vi "_Attenuator Tree.vi"   [LabVIEW 2011]
uses:
  LIB/Attenuator Version.vi
panel:
  # "See Diagram"
types:
  T1 = typedef "OGAB Version.ctl" = cluster{"Version":string, "Build Number":u32, "Build Date/Time":dbl}
  T2 = typedef "Field Record.ctl" = cluster{"ixField":i32, "iSequenceOrder":i32, "sxFieldId":string, "sxSequenceId":string, "sDisplayName":string, "sValue":string, "sUnits":string, "nDataType":T3, "nNextItem":T4, "fSystem":bool, "fSystemValue":bool, "fRequired":bool, "fSetAtTest":bool, "fTestField":bool, "fDeleted":bool, "fIndexed":bool, "fFreeList":bool}
  T3 = typedef "Field DataTypes.ctl" = enum32{"text", "numeric", "list", "timestamp", "boolean"}
  T4 = typedef "Field NextItem.ctl" = enum32{"Reset", "Retain", "Auto-Increment"}
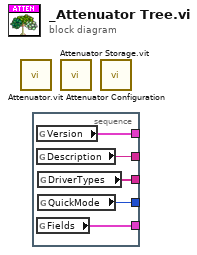
[diagram p0: block diagram]
diagram:
  n1 = call "Attenuator.vit"() -> ()  [unwired: 4 in, 8 out]
  n2 = stacked-sequence {
    tunnel: [w5] -> _
    tunnel: [w4] -> _
    tunnel: [w3] -> _
    tunnel: [w2] -> _
    tunnel: [w1] -> _
    frame #0 {
      n3 = global read "Attenuator Version.vi" "Version"() -> (w5:T1)
      n4 = global read "Attenuator Version.vi" "Description"() -> (w4:string)
      n5 = global read "Attenuator Version.vi" "Fields"() -> (w1:T2[])
      n6 = global read "Attenuator Version.vi" "DriverTypes"() -> (w3:string[])
      n7 = global read "Attenuator Version.vi" "QuickMode"() -> (w2:i32)
    }
  }
  n8 = call "Attenuator Storage.vit"() -> ()  [unwired: 4 in, 8 out]
  n9 = call "Attenuator Configuration.vi"() -> ()  [unwired: 5 in, 7 out]
